vi "ShutDown.vi"(8 "error in (no error)":errorcluster, 11 "TCP_Server in":refnum<class "TCP_Server.lvclass">) -> (0 "error out":errorcluster, 3 "TCP_Server out":refnum<class "TCP_Server.lvclass">)   [LabVIEW 2023, in "TCP_Server.lvlib" / "TCP_Server.lvclass"]
uses:
  TCP_Server.lvclass
  TCP_Server.lvclass/TCP_Server.ctl
  <vilib>/ActorFramework/Actor/Actor.lvclass
  <vilib>/ActorFramework/Stop Msg/Stop Msg.lvclass
  C:/Program Files (x86)/National Instruments/LabVIEW 2023/vi.lib/ActorFramework/Actor/Actor.lvclass
  C:/Source/LabVIEW/TCP_server/TCP_Server/TCP_Server/TCP_Server.lvclass
  C:/Source/LabVIEW/TCP_server/SimpleErrorLogger/ApplicationWithErrorLogger/ApplicationWithErrorLogger.lvclass
  C:/Source/LabVIEW/TCP_server/TCP_Client_Window/TCP_ClientWindow_Controller/TCP_ClientWindow_Controller.lvclass
  C:/Source/LabVIEW/TCP_server/TCP_Listener/Connections Controller/Connections Controller.lvclass
  C:/Source/LabVIEW/TCP_server/TCP_Server_Connection_Handler/TCP_Connections_Controller/TCP_Connections_Controller.lvclass
  C:/Source/LabVIEW/TCP_server/TCP_serverGUI/TCP_ServerWithGUI/TCP_ServerWithGUI.lvclass
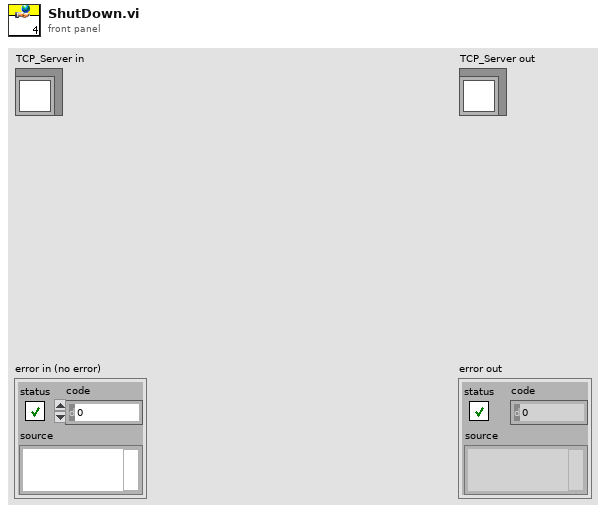
[diagram p1: front panel]
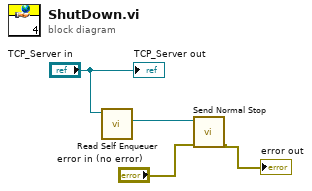
[diagram p0: block diagram]
diagram:
  n1 = call <vilib>:"Read Self Enqueuer.vi"("Actor"="TCP_Server in") -> ("Self Enqueuer"=w3:refnum<class "Message Enqueuer.lvclass">)  [unwired: 10 in]
  n2 = call <vilib>:"Send Normal Stop.vi"("error in (no error)"="error in (no error)", "Message Enqueuer"=w3) -> ("error out"=→"error out":errorcluster)  [unwired: 9 in]
  "TCP_Server out" <- "TCP_Server in"
